vi "Test mupExpr.vi"() -> ()   [LabVIEW 2015]
uses:
  mupExpr/mupExpr.lvclass/mupExpr.ctl
  mupExpr/Eval_MultiVar_SglRes.vi
  mupLib/mupEval.vi
  mupExpr/SetVarVal.vi
  mupLib/mupCheckError.vi
  mupLib/mupLibPath.vi
  mupLib/mupSetVarValue.vi
  <vilib>/Utility/error.llb/Error Cluster From Error Code.vi
  <vilib>/LAVA/AlmostEqual/AlmostEqual_ULPs_DBL.vi
  mupExpr/mupExpr.lvclass
  <vilib>/LAVA/Robust CSV/Robust CSV.lvlib
  <vilib>/LAVA/AlmostEqual/AlmostEqual.lvlib
panel:
  out "Variables":cluster{string, dbl}[](array[cluster]) {"?" format="%_20e"}
  out "NumTests":i32
  out "Failed cases":cluster{string, dbl, "Result":dbl, dbl}[](array[cluster]) {"?" format="%_20e"; "Result" format="%_20e"; "?" format="%_20e"}
  out "NumFails":i32
  in  "Tolerance (ULPs)":u32=100
  out "Test Cases":T1(array[cluster]) {"?" format="%_20e"; "Result" format="%_20e"}
  in  "file path in":path=path "eqTestCases_mupExpr.csv"
  # "Notes:"
  # "muParser evaluates exponents from right to left\na^2^3 = a^(2^3)\nexcel evaluates exponents left to right\na^2^3 = (a^2)^3"
  # "muParser log is base e\n_e^log(a) = a\nexcel log is base 10\n10^log(a) = a"
  # "Expected"
  # "Actual"
  # "Difference"
  # "Expected Result"
  # "Actual Result"
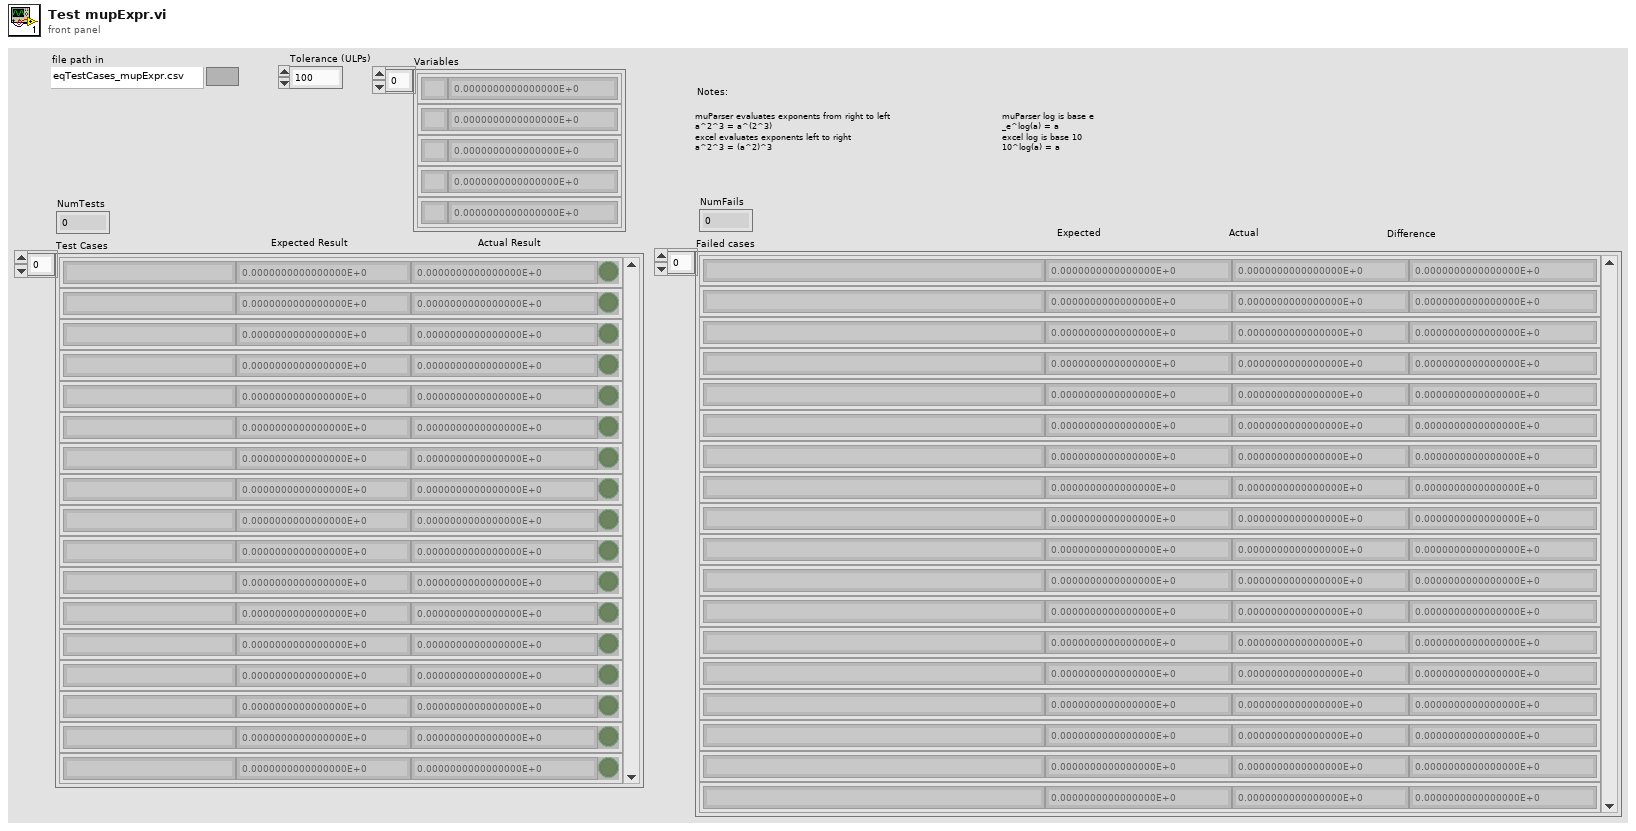
[diagram p1: front panel]
types:
  T1 = cluster{string, dbl, "Result":dbl, "X = Y +/- #ULPs?":bool}[]
  T2 = cluster{string, dbl, "Result":dbl, "X = Y +/- #ULPs?":bool}
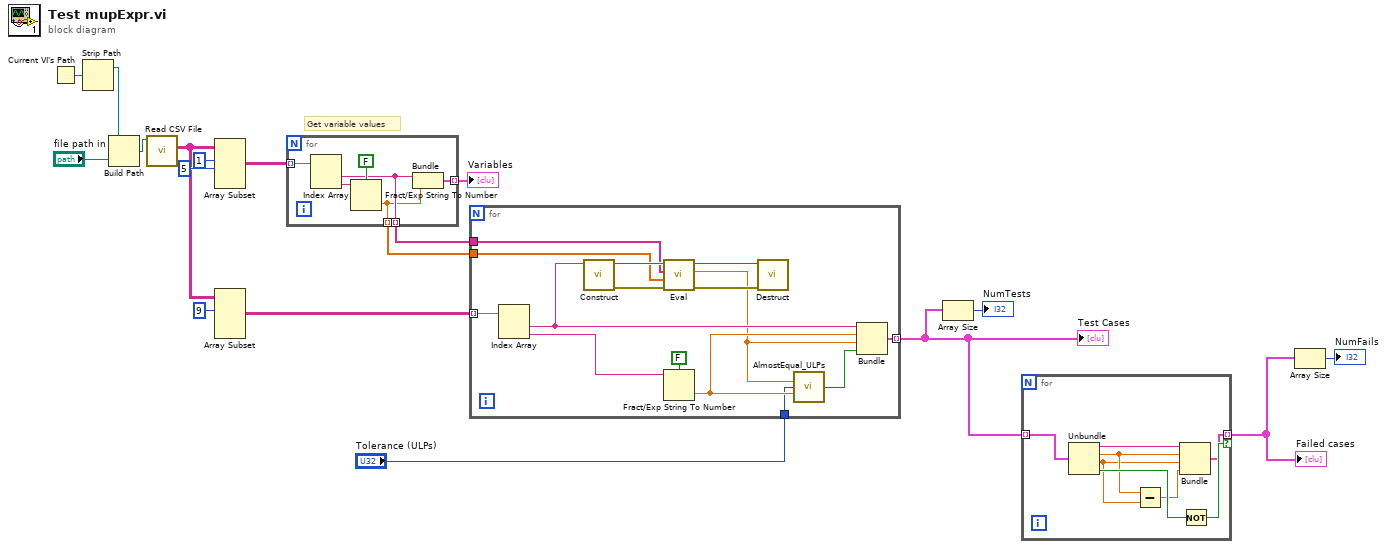
[diagram p0: block diagram]
diagram:
  # "Get variable values"
  n1 = Current VI's Path() -> (path=w4:path)
  n2 = Strip Path(path=w4) -> (stripped path=w2:path)  [unwired: 1 out]
  n3 = Build Path(base path=w2, name or relative path="file path in") -> (appended path=w1:path)
  n4 = call <vilib>:"Read CSV File.vi"("file path in"=w1) -> ("2-D array"=w15:string[][])  [unwired: 8 in, 2 out]
  n5 = Array Subset(array=w15, index (row)=1 ("index"), length (row)=5 ("length")) -> (w16:string[][])  [unwired: 2 in]
  n6 = Array Subset(array=w15, index (row)=9 ("index")) -> (w13:string[][])  [unwired: 3 in]
  n7 = for {
    tunnel: w16 -> [w24] mode=indexing
    tunnel: [w21] -> w5 mode=indexing
    tunnel: [w20] -> w7 mode=indexing
    tunnel: [w19] -> w6 mode=indexing
    n8 = Index Array(array=w24) -> (element #1=w20:string, element #2=w23:string)  [unwired: 2 in]
    n9 = Fract/Exp String To Number(use system decimal point (T)=FALSE, string=w23) -> (number=w19:dbl)  [unwired: 2 in, 1 out]
    n10 = Bundle(w20, w19) -> (w21:cluster{string, dbl})  [unwired: 1 in]
  }
  "Variables" <- w5
  n11 = for {
    tunnel: w13 -> [w35] mode=indexing
    tunnel: [w28] -> w9 mode=indexing
    tunnel: "Tolerance (ULPs)" -> [w27]
    tunnel: w7 -> [w26]
    tunnel: w6 -> [w25]
    n12 = Index Array(array=w35) -> (element #1=w32:string, element #2=w33:string)  [unwired: 2 in]
    n13 = call "Construct.vi"("Expression"=w32) -> ("error out"=w37:errorcluster, "mupExpr out"=w39:refnum<data-value>)  [unwired: 8 in, 1 out]
    n14 = call-poly "Eval.vi"("error in (no error)"=w37, "varValues"=w25, "varNames"=w26, "mupExpr in"=w39) -> ("error out"=w36:errorcluster, "Result"=w30:dbl, "mupExpr out"=w38:refnum<data-value>)  [unwired: 5 in]
    n15 = Fract/Exp String To Number(use system decimal point (T)=FALSE, string=w33) -> (number=w31:dbl)  [unwired: 2 in, 1 out]
    n16 = call "Destruct.vi"("error in (no error)"=w36, "mupExpr in"=w38) -> ()  [unwired: 9 in, 1 out]
    n17 = call-poly <vilib>:"AlmostEqual_ULPs.vi"("X"=w30, "Tolerance (5 ULPs)"=w27, "Y"=w31) -> ("X = Y +/- #ULPs?"=w29:bool)  [unwired: 12 in]
    n18 = Bundle(w32, w31, "Result"=w30, "X = Y +/- #ULPs?"=w29) -> (w28:T2)  [unwired: 1 in]
  }
  "Test Cases" <- w9
  n19 = Array Size(array=w9) -> (size(s)=→"NumTests":i32)
  n20 = for {
    tunnel: w9 -> [w47] mode=indexing
    tunnel: [w40] -> w11 mode=indexing if=w45
    n21 = Unbundle(w47) -> (w44:string, w43:dbl, "Result"=w42:dbl, "X = Y +/- #ULPs?"=w46:bool)
    n22 = Subtract(x=w43, y=w42) -> (x-y=w41:dbl)
    n23 = Bundle(w44, w43, "Result"=w42, w41) -> (w40:cluster{string, dbl, "Result":dbl, dbl})  [unwired: 1 in]
    n24 = Not(x=w46) -> (.not. x?=w45:bool)
  }
  "Failed cases" <- w11
  n25 = Array Size(array=w11) -> (size(s)=→"NumFails":i32)
